vi "Create Knock Cylinder Tree Layout.vi"(8 "error in (no error)":errorcluster, 10 "cylinder name":string, 11 "Section Ptr":T1 format="%.0x") -> (0 "error out":errorcluster, 3 "Section Ptr dup":T1 format="%.0x")   [LabVIEW 2017, in "Engine Simulation Toolkit System Explorer.lvlib"]
uses:
  Engine Simulation Toolkit System Explorer.lvlib
  <vilib>/NI Veristand/Custom Device API/Custom Device Item Ref.ctl
  <vilib>/NI Veristand/Custom Device API/Custom Device Channel Type.ctl
  Shared/Constants and GUIDs.vi
  Shared/Properties.vi
  <vilib>/NI Veristand/Custom Device API/Set Item Property (String).vi
  Shared/Engine Simulation Toolkit Shared.lvlib
  <vilib>/NI Veristand/Custom Device API/Custom Device API.lvlib
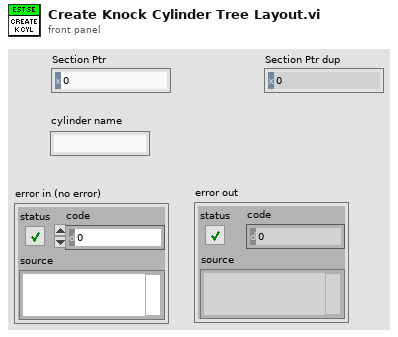
[diagram p1: front panel]
types:
  T1 = typedef "Custom Device API.lvlib/Custom Device Item Ref.ctl" = u64
  T2 = typedef "Custom Device API.lvlib/Custom Device Channel Type.ctl" = enum16{"Input", "Output"}
  T3 = typedef "Engine Simulation Toolkit Shared.lvlib/Channel.ctl" = cluster{"Name":string, "Units":string, "Default":dbl, "Description":string, "Scalable":bool}
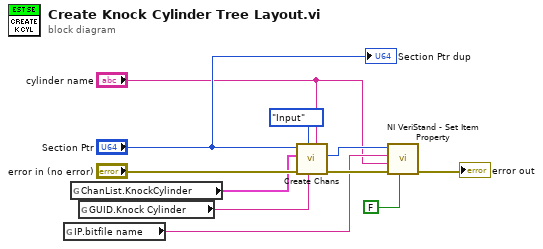
[diagram p0: block diagram]
diagram:
  n1 = global read "Properties.vi" "IP.bitfile name"() -> (w3:string)
  n2 = global read "Constants and GUIDs.vi" "ChanList.KnockCylinder"() -> (w9:T3[])
  n3 = global read "Constants and GUIDs.vi" "GUID.Knock Cylinder"() -> (w8:string)
  n4 = call "Create Chans.vi"("New Section Name (none)"="cylinder name", "new section GUID (\"\":del prot)"=w8, "Type"=Custom_Device_Channel_Type."Input", "error in (no error)"="error in (no error)", "Channels"=w9, "Section Ptr"="Section Ptr") -> ("error out"=w6:errorcluster, "new section ref"=w4:T1)  [unwired: 2 in, 2 out]
  n5 = call-poly <vilib>:"NI VeriStand - Set Item Property.vi"("Binary String (T)"=FALSE, "error in (no error)"=w6, "Value"="cylinder name", "Property Name"=w3, "Item Ref in"=w4) -> ("error out"=→"error out":errorcluster)  [unwired: 4 in, 2 out]
  "Section Ptr dup" <- "Section Ptr"
